vi "Loop Wrapper.vi"(9 "Error Queue":refnum<queue>, 10 "Helper Loop Queue":refnum<queue>, 11 "Helper Loop in":refnum<class "Event Actor.lvclass">) -> ()   [LabVIEW 2021, in "Event Actor.lvclass"]
uses:
  Event Actor.lvclass
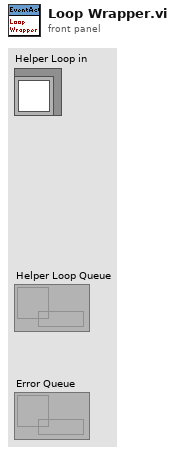
[diagram p1: front panel]
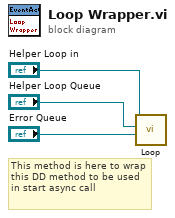
[diagram p0: block diagram]
diagram:
  # "This method is here to wrap this DD method to be used in start async call"
  n1 = call-dynamic "Loop.vi"("Error Queue"="Error Queue", "Helper Loop Queue"="Helper Loop Queue", "Helper Loop in"="Helper Loop in") -> ()  [unwired: 9 in]
